vi "main.vi"() -> ()   [LabVIEW 2017]
uses:
  <vilib>/DAQmx/read.llb/DAQmx Read (Analog 2D DBL NChan NSamp).vi
  <vilib>/Analysis/baseanly.llb/Mean (DBL).vi
  <vilib>/DAQmx/create/channels.llb/DAQmx Create Channel (AI-Temperature-Thermocouple).vi
  <vilib>/DAQmx/create/channels.llb/DAQmx Create Channel (AI-Voltage-Basic).vi
  <vilib>/DAQmx/configure/timing.llb/DAQmx Timing (Sample Clock).vi
  <vilib>/DAQmx/miscellaneous.llb/DAQmx Fill In Error Info.vi
  <vilib>/Analysis/NI_AALBase.lvlib
panel:
  out "Torque graph":dbl[](graph)
  in  "torque_cell_channels":tag
  in  "temperature_channels":tag
  out "Speed":dbl(knob) scale=0.0..4000.0
  out "UUT":dbl(slide) scale=0.0..100.0
  out "Oil Tank":dbl(slide) scale=0.0..100.0
  out "Room":dbl(slide) scale=0.0..100.0
  in  "stop":bool
  # "1/min"
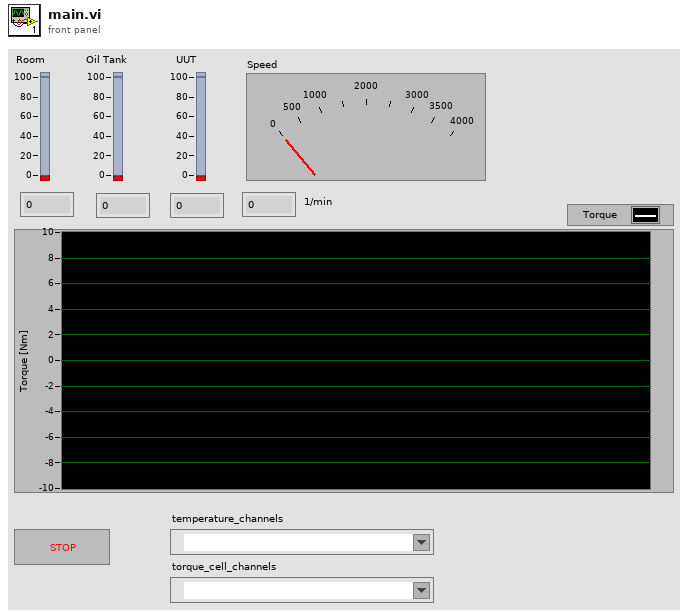
[diagram p1: front panel]
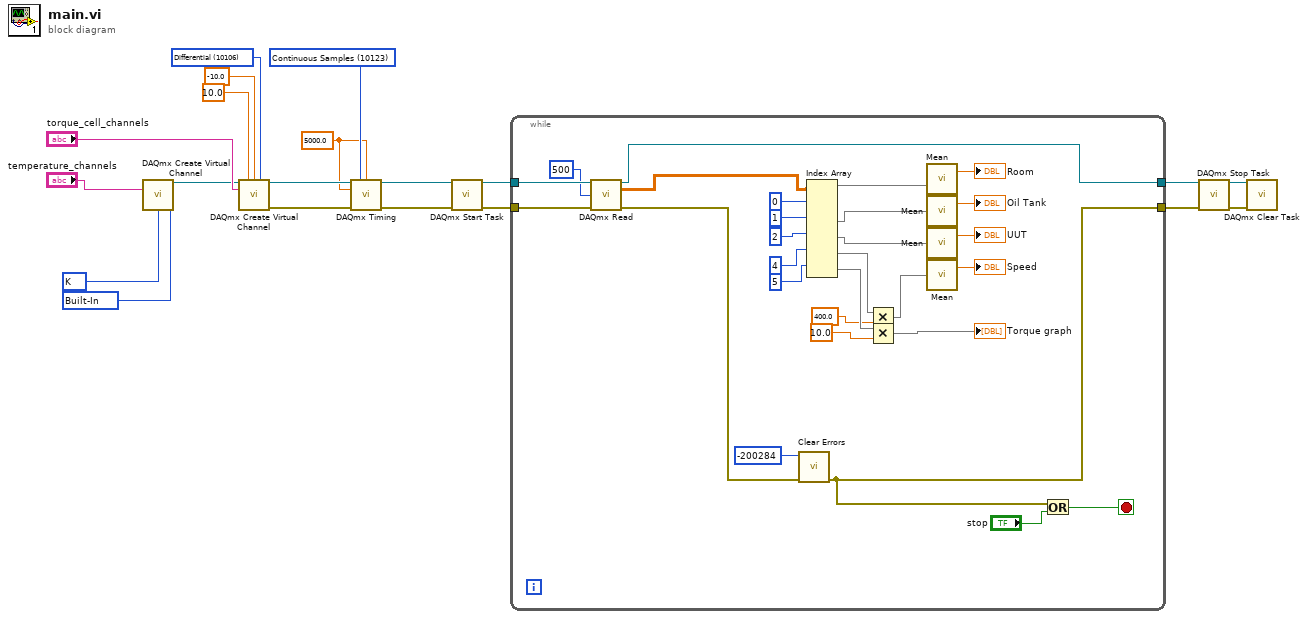
[diagram p0: block diagram]
diagram:
  w4 = 10123 items=["Finite Samples"=10178, "Continuous Samples"=10123, "Hardware Timed Single Point"=12522] ("sample mode")
  w3 = 5000.0 ("rate")
  w13 = 10106 items=["Default"=-1, "RSE"=10083, "NRSE"=10078, "Differential"=10106, "Pseudodifferential"=12529] ("input terminal configuration")
  w16 = 10200 items=["Built-In"=10200, "Constant Value"=10116, "Channel"=10113] ("cjc source")
  w17 = 10073 items=["J"=10072, "K"=10073, "N"=10077, "R"=10082, "S"=10085, "T"=10086, "B"=10047, "E"=10055] ("thermocouple type")
  n1 = call-poly <vilib>:"DAQmx Create Virtual Channel.vi"("physical channels"="temperature_channels", "cjc source"=w16, "thermocouple type"=w17) -> ("task out"=w18:refnum<k21>)  [unwired: 11 in, 1 out]
  n2 = call-poly <vilib>:"DAQmx Create Virtual Channel.vi"("task in"=w18, "maximum value"=10.0, "minimum value"=-10.0, "input terminal configuration"=w13, "physical channels"="torque_cell_channels") -> ("task out"=w6:refnum<k21>, "error out"=w5:errorcluster)  [unwired: 9 in]
  n3 = call-poly <vilib>:"DAQmx Timing.vi"("task/channels in"=w6, "sample mode"=w4, "samples per channel"=w3, "rate"=w3, "error in"=w5) -> ("task out"=w1:refnum<k21>, "error out"=w2:errorcluster)  [unwired: 9 in]
  n4 = call <vilib>:"DAQmx Start Task.vi"("task/channels in"=w1, "error in"=w2) -> ("task out"=w12:refnum<k21>, "error out"=w11:errorcluster)  [unwired: 12 in]
  n5 = while {
    tunnel: w12 -> [w48]
    tunnel: w11 -> [w47]
    tunnel: [w41] -> w10
    tunnel: [w36] -> w7
    stop <- w39 stop-if-true
    n6 = call-poly <vilib>:"DAQmx Read.vi"("task/channels in"=w48, "number of samples per channel"=500, "error in"=w47) -> ("task out"=w41:refnum<k21>, "data"=w23:dbl[][], "error out"=w38:errorcluster)  [unwired: 10 in]
    n7 = call <vilib>:"Clear Errors.vi"("error in (no error)"=w38, "specific error code to clear (0: all)"=-200284) -> ("error out"=w36:errorcluster)  [unwired: 4 in, 1 out]
    n8 = Index Array(array=w23, index (row) #1=0 ("index"), index (row) #2=1 ("index"), index (row) #3=2 ("index"), index (row) #4=4 ("index"), index (row) #5=5 ("index")) -> (element #1=w31:dbl[], element #2=w29:dbl[], element #3=w27:dbl[], element #4=w33:dbl[], element #5=w34:dbl[])  [unwired: 5 in]
    n9 = Multiply(x=w33, y=400.0) -> (x*y=w25:dbl[])
    n10 = Multiply(x=w34, y=10.0) -> (x*y=→"Torque graph":dbl[])
    n11 = call-poly <vilib>:"Mean.vi"("X"=w31) -> ("mean"=→"Room":dbl)  [unwired: 1 out]
    n12 = call-poly <vilib>:"Mean.vi"("X"=w29) -> ("mean"=→"Oil Tank":dbl)  [unwired: 1 out]
    n13 = call-poly <vilib>:"Mean.vi"("X"=w27) -> ("mean"=→"UUT":dbl)  [unwired: 1 out]
    n14 = call-poly <vilib>:"Mean.vi"("X"=w25) -> ("mean"=→"Speed":dbl)  [unwired: 1 out]
    n15 = Or(x=w36, y="stop") -> (x .or. y?=w39:bool)
  }
  n16 = call <vilib>:"DAQmx Stop Task.vi"("task/channels in"=w10, "error in"=w7) -> ("task out"=w9:refnum<k21>, "error out"=w8:errorcluster)  [unwired: 12 in]
  n17 = call <vilib>:"DAQmx Clear Task.vi"("task in"=w9, "error in"=w8) -> ()  [unwired: 13 in, 1 out]
